vi "testAddStatesToQueueReentrant.vi"(8 "error in (no error)":errorcluster, 11 "testStateMachineUtilities in":refnum<class "testStateMachineUtilities.lvclass">) -> (0 "error out":errorcluster, 3 "testStateMachineUtilities out":refnum<class "testStateMachineUtilities.lvclass">)   [LabVIEW 2013, in "testStateMachineUtilities.lvclass"]
uses:
  testStateMachineUtilities.lvclass
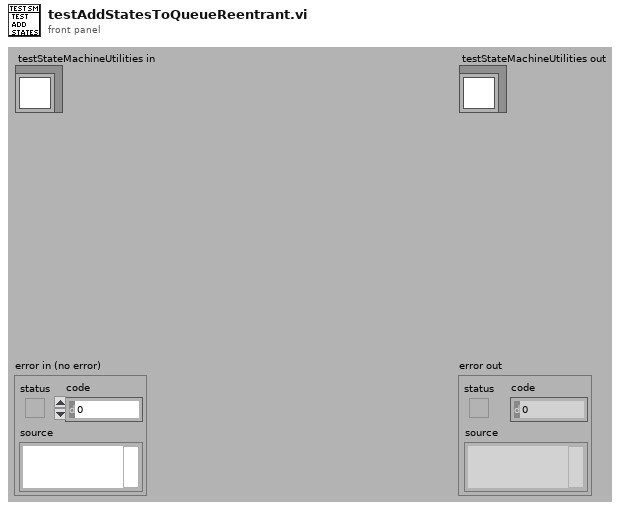
[diagram p1: front panel]
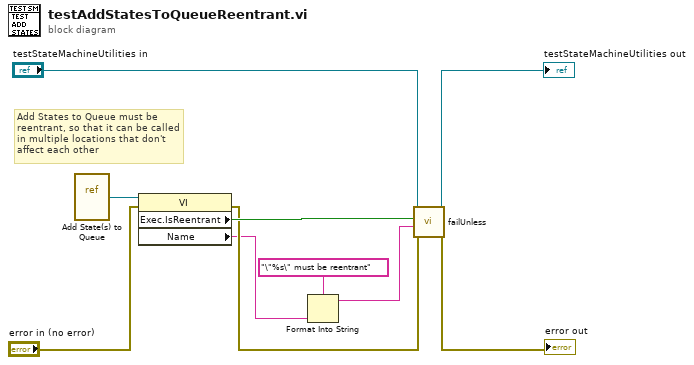
[diagram p0: block diagram]
diagram:
  # "Add States to Queue must be reentrant, so that it can be called in multiple locations that don't affect each other"
  n1 = vi-ref "Add State(s) to Queue.vi"() -> (w7:refnum<vi>)
  n2 = property class="VI"(reference=w7, error in="error in (no error)") -> (error out=w2:errorcluster, "Exec.IsReentrant"=w6:bool, "Name"=w1:string)  [unwired: 1 out]
  n3 = Format Into String(format string="\"%s\" must be reentrant", w1) -> (resulting string=w5:string)  [unwired: 2 in, 1 out]
  n4 = call-dynamic "failUnless.vi"("error in (no error)"=w2, "message (\"\")"=w5, "pass"=w6, "TestCase in"="testStateMachineUtilities in") -> ("error out"=→"error out":errorcluster, "TestCase out"=→"testStateMachineUtilities out":refnum<class "testStateMachineUtilities.lvclass">)  [unwired: 6 in]
